vi "STS_Cal_IL_Merge.vi"(8 "错误输入（无错误）":errorcluster, 10 "type":i32(ring) items=["MPM_10"=0, "MPM_211"=1, "MPM_212"=2, "MPM_213"=3, "MPM_215"=5], 11 ".NET引用句柄输入":refnum<k24>) -> (0 "error out":errorcluster, 3 "引用输出":refnum<k24>)   [LabVIEW 2017]
doc: "Process ranges merge"
uses:
  D:/test/PDLSTS/LV_PDL LvVer17.0/LV_PDL_x86/DLL/STSProcess.dll
  DLL/STSProcess.dll
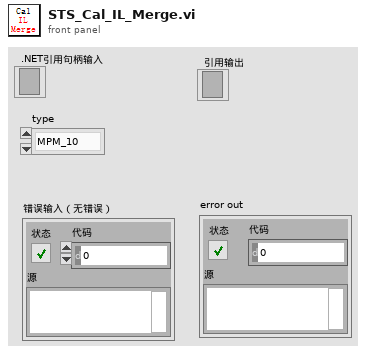
[diagram p1: front panel]
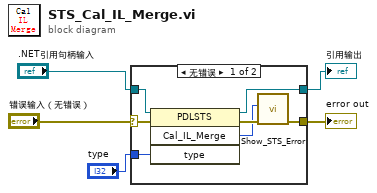
[diagram p0: block diagram]
diagram:
  n1 = case shown="无错误" "错误输入（无错误）" {
    selector: "错误输入（无错误）" -> [w11 w14]
    tunnel: ".NET引用句柄输入" -> [w12 w13]
    tunnel: [w8 w14] -> w3
    tunnel: [w7 w13] -> w2
    tunnel: "type" -> [w6 _]
    frame No Error {
      n2 = invoke class="PDLSTS" method="Cal_IL_Merge"(reference=w12, error in=w11, "type"=w6) -> (reference out=w7:refnum<k24>, error out=w10:errorcluster, "Cal_IL_Merge"=w9:i32)  [unwired: 1 in, 1 out]
      n3 = call "Show_STS_Error.vi"("error in (no error)"=w10, "Error"=w9) -> ("error out"=w8:errorcluster)  [unwired: 9 in]
    }
    frame Error {
    }
  }
  "error out" <- w3
  "引用输出" <- w2
